vi "Connect.vi"(11 "Device Serial Number":string) -> (1 "Handle":u32, 3 "FT_Status":u32(ring) items=["FT_OK", "FT_INVALID_HANDLE", "FT_DEVICE_NOT_FOUND", "FT_DEVICE_NOT_OPENED", "FT_IO_ERROR", "FT_INSUFFICIENT_RESOURCES", "FT_INVALID_PARAMETER", "FT_INVALID_BAUD_RATE", "FT_DEVICE_NOT_OPENED_FOR_ERASE", "FT_DEVICE_NOT_OPENED_FOR_WRITE", "FT_FAILED_TO_WRITE_DEVICE", "FT_EEPROM_READ_FAILED", "FT_EEPROM_WRITE_FAILED", "FT_EEPROM_ERASE_FAILED", "FT_EEPROM_NOT_PRESENT", "FT_EEPROM_NOT_PROGRAMMED", "FT_INVALID_ARGS", "FT_NOT_SUPPORTED", "FT_OTHER_ERROR"])   [LabVIEW 2013]
panel:
  in  "Index":i32
  out "Count 3":i32
  out "Count 2":i32
  out "Count 1":i32
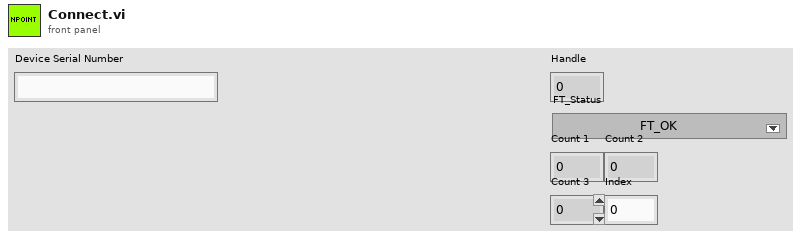
[diagram p1: front panel]
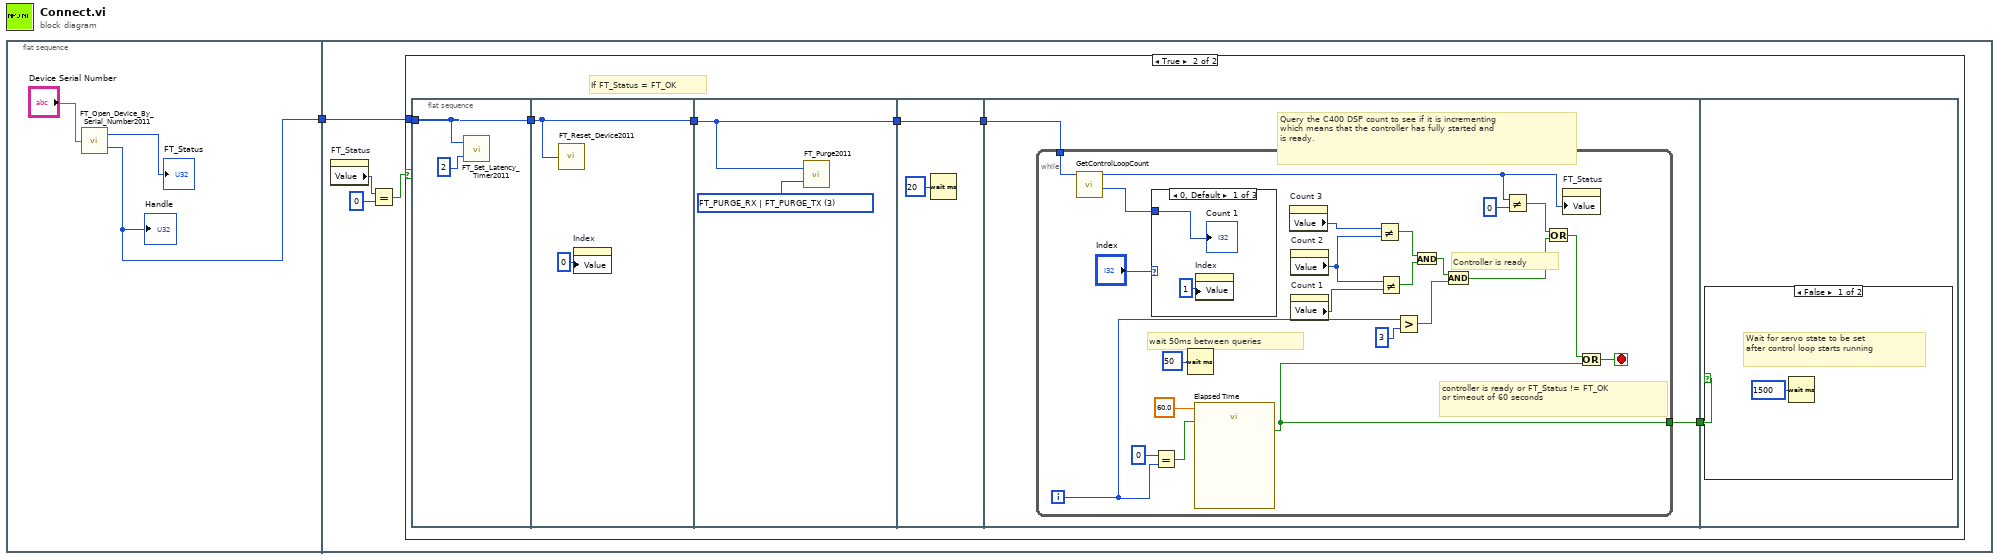
[diagram p0: block diagram]
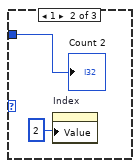
[diagram p3: hidden frame]
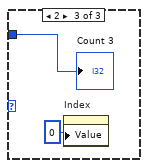
[diagram p4: hidden frame]
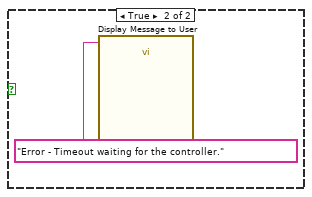
[diagram p5: hidden frame]
diagram:
  n1 = flat-sequence {
    tunnel: [w2] -> w1
    tunnel: w1 -> [w5]
    frame #0 {
      n2 = call "FT_Open_Device_By_Serial_Number2011.vi"("Device Serial Number"="Device Serial Number") -> ("FT_Status"=→"FT_Status":u32, "Handle"=w2:u32)
      "Handle" <- w2
    }
    frame #1 {
      n3 = property on="FT_Status" class="Ring (strict)"() -> ("Value"=w7:u32)  [unwired: 2 in, 2 out]
      n4 = Equal?(x=w7, y=u32 0) -> (x = y?=w8:bool)
      n5 = case shown="True" w8 {
        tunnel: w5 -> [_ w14]
        frame False {
        }
        frame True {
          # "If FT_Status = FT_OK"
          n6 = flat-sequence {
            tunnel: w14 -> [w16]
            tunnel: [w16] -> w9
            tunnel: [w18] -> w13
            tunnel: w9 -> [w18]
            tunnel: w13 -> [w19]
            tunnel: [w19] -> w11
            tunnel: [w21] -> w12
            tunnel: w11 -> [w21]
            tunnel: w12 -> [w24]
            tunnel: [w23] -> w10
            tunnel: w10 -> [w54]
            frame #0 {
              n7 = call "FT_Set_Latency_Timer2011.vi"("Latency Timer Value"=u8 2, "Handle"=w16) -> ()  [unwired: 1 out]
            }
            frame #1 {
              n8 = call "FT_Reset_Device2011.vi"("Handle"=w18) -> ()  [unwired: 1 out]
              n9 = property on="Index" class="DigNum (strict)"("Value"=0 ("Index")) -> ()  [unwired: 2 in, 2 out]
            }
            frame #2 {
              w20 = u32 3 items=["FT_PURGE_RX"=1, "FT_PURGE_TX"=2, "FT_PURGE_RX | FT_PURGE_TX"=3] ("Purge Flags")
              n10 = call "FT_Purge2011.vi"("Purge Flags"=w20, "Handle"=w19) -> ()  [unwired: 1 out]
            }
            frame #3 {
              n11 = Wait (ms)(milliseconds to wait=u32 20) -> ()  [unwired: 1 out]
            }
            frame #4 {
              # "Query the C400 DSP count to see if it is incrementing\nwhich means that the controller has fully started and \nis ready."
              n12 = while {
                tunnel: w24 -> [w47]
                tunnel: [w25] -> w23
                i -> [w28]
                stop <- w26 stop-if-true
                # "wait 50ms between queries"
                # "controller is ready or FT_Status != FT_OK\nor timeout of 60 seconds"
                # "Controller is ready"
                n13 = call "GetControlLoopCount.vi"("Handle"=w47) -> ("FT_Status"=w32:u32, "Control Loop Count"=w44:i32)  [unwired: 8 in]
                n14 = case shown="0, Default" "Index" {
                  tunnel: w44 -> [w49 w51 w53]
                  frame 0, Default {
                    n15 = property on="Index" class="DigNum (strict)"("Value"=1 ("Index")) -> ()  [unwired: 2 in, 2 out]
                    "Count 1" <- w49
                  }
                  frame 1 {
                    n16 = property on="Index" class="DigNum (strict)"("Value"=2 ("Index")) -> ()  [unwired: 2 in, 2 out]
                    "Count 2" <- w51
                  }
                  frame 2 {
                    n17 = property on="Index" class="DigNum (strict)"("Value"=0 ("Index")) -> ()  [unwired: 2 in, 2 out]
                    "Count 3" <- w53
                  }
                }
                n18 = Equal?(x=0, y=w28) -> (x = y?=w30:bool)
                n19 = Wait (ms)(milliseconds to wait=u32 50) -> ()  [unwired: 1 out]
                n20 = call "Elapsed Time"("Time Target (s)"=60.0, "Reset"=w30) -> ("Time has Elapsed"=w25:bool)  [unwired: 10 in, 7 out]
                n21 = property on="Count 3" class="DigNum (strict)"() -> ("Value"=w42:i32)  [unwired: 2 in, 2 out]
                n22 = property on="Count 2" class="DigNum (strict)"() -> ("Value"=w40:i32)  [unwired: 2 in, 2 out]
                n23 = property on="Count 1" class="DigNum (strict)"() -> ("Value"=w41:i32)  [unwired: 2 in, 2 out]
                n24 = Not Equal?(x=w42, y=w40) -> (x != y?=w39:bool)
                n25 = Not Equal?(x=w40, y=w41) -> (x != y?=w38:bool)
                n26 = Greater?(x=w28, y=3) -> (0:w37:bool)
                n27 = And(x=w39, y=w38) -> (x .and. y?=w36:bool)
                n28 = And(x=w36, y=w37) -> (x .and. y?=w34:bool)
                n29 = Not Equal?(x=w32, y=u32 0) -> (x != y?=w33:bool)
                n30 = Or(x=w33, y=w34) -> (x .or. y?=w27:bool)
                n31 = property on="FT_Status" class="Ring (strict)"("Value"=w32) -> ()  [unwired: 2 in, 2 out]
                n32 = Or(x=w27, y=w25) -> (x .or. y?=w26:bool)
              }
            }
            frame #5 {
              n33 = case shown="False" w54 {
                frame False {
                  # "Wait for servo state to be set\nafter control loop starts running"
                  n34 = Wait (ms)(milliseconds to wait=u32 1500) -> ()  [unwired: 1 out]
                }
                frame True {
                  n35 = call "Display Message to User"("Message"="Error - Timeout waiting for the controller.") -> ()  [unwired: 9 in, 2 out]
                }
              }
            }
          }
        }
      }
    }
  }
